vi "Test Flag Get and Set.vi"(8 "error in (no error)":errorcluster, 11 "TestCase in":refnum<class "Debug Tests.lvclass">) -> (0 "error out":errorcluster, 3 "TestCase out":refnum<class "Debug Tests.lvclass">)   [LabVIEW 2017, in "Debug Tests.lvclass"]
uses:
  Debug Tests.lvclass
  Engine/Classes/Debug/FIFO Flags/FIFO Flags.lvclass
  Engine/Classes/Debug/Debug Flags/Debug Flags.lvclass
  Engine/Classes/Debug/FIFO Flags/FIFO Flags.lvclass/FIFO Flags.ctl
  Engine/Classes/Debug/Debug Flags/Debug Flags.lvclass/Debug Flags.ctl
  <vilib>/addons/_JKI Toolkits/VI Tester/TestCase.llb/TestCase.lvclass
  C:/Program Files (x86)/National Instruments/LabVIEW 2017/vi.lib/addons/_JKI Toolkits/VI Tester/TestCase.llb/TestCase.lvclass
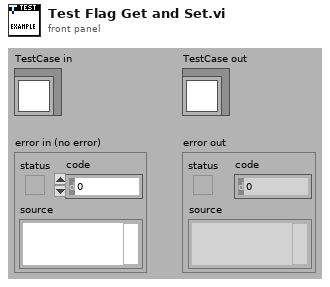
[diagram p1: front panel]
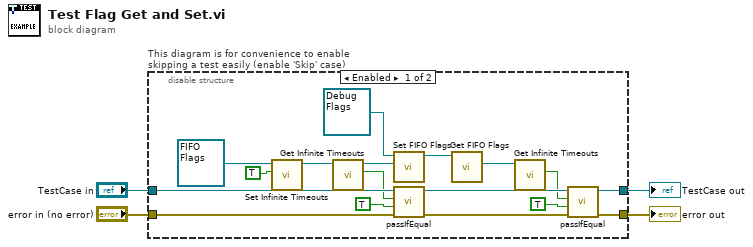
[diagram p0: block diagram]
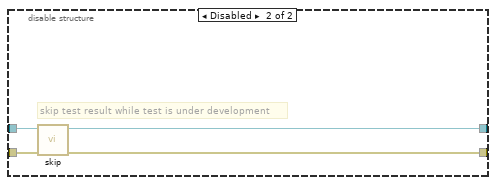
[diagram p2: hidden frame]
diagram:
  n1 = disable-structure "This diagram is for convenience to enable skipping a test easily (enable 'Skip' case)" shown="Enabled" {
    disable-tunnel: "TestCase in" -> [w16 w25]
    disable-tunnel: [w7 w23] -> w1
    disable-tunnel: [w9 w24] -> w3
    disable-tunnel: "error in (no error)" -> [w21 w22]
    frame Enabled {
      n2 = call "Set Infinite Timeouts.vi"("infinite timeouts"=TRUE, "FIFO Debug Flags in"=refnum<class "FIFO Flags.lvclass"> refnum) -> ("FIFO Debug Flags out"=w19:refnum<class "FIFO Flags.lvclass">)  [unwired: 9 in]
      n3 = call "Get Infinite Timeouts.vi"("FIFO Debug Flags in"=w19) -> ("infinite timeouts"=w15:bool, "FIFO Debug Flags out"=w12:refnum<class "FIFO Flags.lvclass">)  [unwired: 9 in]
      n4 = call "Set FIFO Flags.vi"("FIFO"=w12, "Debug Flags in"=refnum<class "Debug Flags.lvclass"> refnum) -> ("Debug Flags out"=w13:refnum<class "Debug Flags.lvclass">)  [unwired: 9 in]
      n5 = call-dynamic "passIfEqual.vi"("error in (no error)"=w21, "y"=TRUE ("infinite timeouts"), "x"=w15, "TestCase in"=w16) -> ("error out"=w17:errorcluster, "TestCase out"=w8:refnum<class "Debug Tests.lvclass">)  [unwired: 6 in]
      n6 = call "Get FIFO Flags.vi"("Debug Flags in"=w13) -> ("FIFO"=w10:refnum<class "FIFO Flags.lvclass">)  [unwired: 9 in, 1 out]
      n7 = call "Get Infinite Timeouts.vi"("FIFO Debug Flags in"=w10) -> ("infinite timeouts"=w6:bool)  [unwired: 9 in, 1 out]
      n8 = call-dynamic "passIfEqual.vi"("error in (no error)"=w17, "y"=TRUE ("infinite timeouts"), "x"=w6, "TestCase in"=w8) -> ("error out"=w9:errorcluster, "TestCase out"=w7:refnum<class "Debug Tests.lvclass">)  [unwired: 6 in]
    }
    frame Disabled {
      # "skip test result while test is under development"
      n9 = call <vilib>:"skip.vi"("error in (no error)"=w22, "TestCase in"=w25) -> ("error out"=w24:errorcluster, "TestCase out"=w23:refnum<class "Debug Tests.lvclass">)  [unwired: 8 in]
    }
  }
  "error out" <- w3
  "TestCase out" <- w1
